vi "Initiate drain sweep and perform measurement.vi"(10 "Drain sweep":T1, 11 "VISA Refnum in":refnum<visa-resource-name>) -> (0 "error out":errorcluster, 1 "Voltage":dbl[](array[numeric]), 2 "Current":dbl[](array[numeric]), 3 "VISA Refnum out":refnum<visa-resource-name>)   [LabVIEW 2021]
uses:
  <instrlib>/Keithley 2450/Keithley 2450.lvlib
  <instrlib>/Keithley 2450/Public/Data/Read (Multiple Points).vi
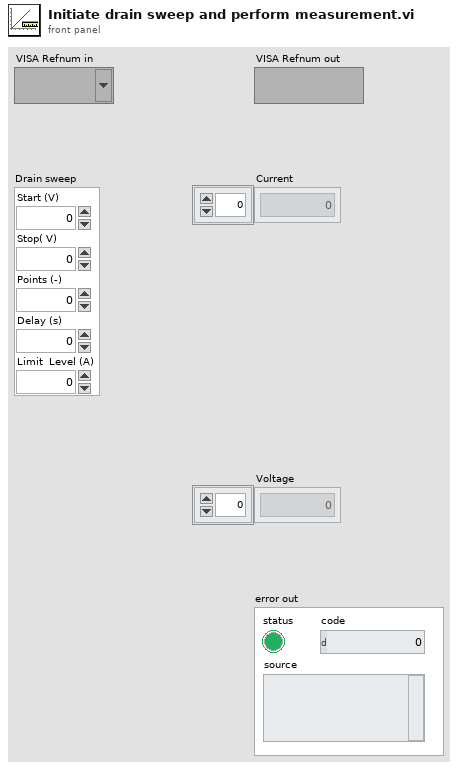
[diagram p1: front panel]
types:
  T1 = cluster{"Start (V) ":dbl, "Stop( V) ":dbl, "Points (-)":u32, "Delay (s)":dbl, "Limit  Level (A)":dbl}
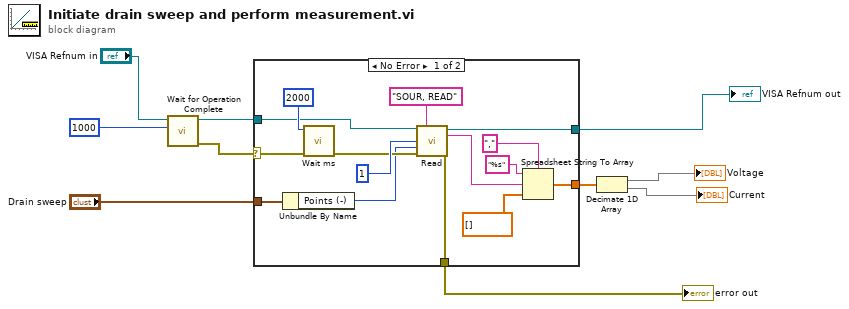
[diagram p0: block diagram]
diagram:
  n1 = call <instrlib>:"Wait for Operation Complete.vi"("Timeout (10000 ms)"=u32 1000, "VISA resource name"="VISA Refnum in") -> ("error out"=w1:errorcluster, "VISA resource name out"=w3:refnum<visa-resource-name>)  [unwired: 8 in]
  n2 = case shown="No Error" w1 {
    selector: w1 -> [w11 _]
    tunnel: [w24 _] -> w8
    tunnel: [w16 _] -> w7
    tunnel: [w15 w26] -> w6
    tunnel: "Drain sweep" -> [w13 _]
    tunnel: w3 -> [w12 w26]
    frame No Error {
      n3 = Unbundle By Name(w13) -> ("Points (-)"=w14:u32)
      n4 = call "Wait ms.vi"("error in (no error)"=w11, "milliseconds to wait"=u32 2000) -> ("error in (no error) 2"=w21:errorcluster)  [unwired: 9 in]
      n5 = call-poly <instrlib>:"Read.vi"("VISA resource name"=w12, "Buffer Elements"="SOUR, READ", "Start Index (1)"=u32 1, "End Index (1)"=w14, "error in (no error)"=w21) -> ("VISA resource name out"=w15:refnum<visa-resource-name>, "Data out"=w23:string, "error out"=w24:errorcluster)  [unwired: 8 in]
      n6 = Spreadsheet String To Array(delimiter (Tab)=",", format string="%s", spreadsheet string=w23, array type (2D Dbl)=dbl[] []) -> (array=w16:dbl[])
    }
    frame Error {
    }
  }
  "error out" <- w8
  "VISA Refnum out" <- w6
  n7 = Decimate 1D Array(w7) -> (→"Voltage":dbl[], →"Current":dbl[])
